vi "LSMcontroller_v57.vi"() -> ()   [LabVIEW 2015] (continued)
                n2498 = property on="Sampling rate" class="DigNum (strict)"("Visible"=FALSE, "DisabledEnum"=T8."Disabled" ("Disabled")) -> ()  [unwired: 2 in, 2 out]
                n2499 = property on="Pel" class="DigNum (strict)"("Visible"=w5442, "DisabledEnum"=w5443) -> ()  [unwired: 2 in, 2 out]
                n2500 = property on="bin" class="DigNum (strict)"("Visible"=w5442, "DisabledEnum"=w5443) -> ()  [unwired: 2 in, 2 out]
                n2501 = call "2pparameters.vi"("Params in"=w5453, "command"="set") -> ()  [unwired: 1 out]
              }
              frame "Lifetime (point)" {
                w5476 = T8."Enabled" ("Disabled")
                w5475 = TRUE ("Visible")
                n2502 = property on="Pel" class="DigNum (strict)"("Visible"=w5475, "DisabledEnum"=w5476) -> ()  [unwired: 2 in, 2 out]
                n2503 = property on="bin" class="DigNum (strict)"("Visible"=w5475, "DisabledEnum"=w5476) -> ()  [unwired: 2 in, 2 out]
                n2504 = property on="ttt" class="Enum (strict)"("Visible"=FALSE) -> ()  [unwired: 2 in, 2 out]
                n2505 = local write "Zscantab"(enum32{"withzscan", "withoutzscan", "lifetime"}."lifetime" ("Zscantab")) -> ()
                n2506 = local write "graphtab"(T6."Lifetime" ("graphtab")) -> ()
                n2507 = local write "Meastab"(enum32{"X-Y Image", "Linescan", "Timetrace"}."Timetrace" ("Meastab")) -> ()
                n2508 = call "lifetimeparameters.vi"("command"="get") -> ("Params out"=w5483:T21)  [unwired: 1 in]
                n2509 = Unbundle By Name(w5483) -> ("initialized"=w5484:bool)
                n2510 = property on="srateAODOtt" class="DigNum (strict)"("Visible"=TRUE, "DisabledEnum"=T8."Enabled" ("Disabled")) -> ()  [unwired: 2 in, 2 out]
                n2511 = case shown="False" w5484 {
                  frame False {
                    n2512 = property on="Init" class="Bool (strict)"("Visible"=TRUE, "DisabledEnum"=T8."Enabled" ("Disabled")) -> ()  [unwired: 2 in, 2 out]
                    n2513 = property on="Start" class="Bool (strict)"("Visible"=FALSE, "DisabledEnum"=T8."Disabled and Grayed Out" ("Disabled")) -> ()  [unwired: 2 in, 2 out]
                  }
                  frame True {
                  }
                }
                n2514 = property on="Sampling rate" class="DigNum (strict)"("Visible"=FALSE, "DisabledEnum"=T8."Disabled" ("Disabled")) -> ()  [unwired: 2 in, 2 out]
              }
              frame "Lifetime (scan)" {
                w5493 = T8."Disabled" ("Disabled")
                w5492 = FALSE ("Visible")
                n2515 = call "lifetimeparameters.vi"("command"="get") -> ("Params out"=w5505:T21)  [unwired: 1 in]
                n2516 = local write "graphtab"(T6."image" ("graphtab")) -> ()
                n2517 = local write "Save tab"(enum32{"withsave", "withoutsave"}."withsave" ("Save tab")) -> ()
                n2518 = local write "Meastab"(enum32{"X-Y Image", "Linescan", "Timetrace"}."X-Y Image" ("Meastab")) -> ()
                n2519 = local write "Zscantab"(enum32{"withzscan", "withoutzscan", "lifetime"}."lifetime" ("Zscantab")) -> ()
                n2520 = Unbundle By Name(w5505) -> ("initialized"=w5504:bool)
                n2521 = property on="ttt" class="Enum (strict)"("Visible"=FALSE) -> ()  [unwired: 2 in, 2 out]
                n2522 = property on="refreshtime" class="DigNum (strict)"("Visible"=FALSE, "DisabledEnum"=T8."Disabled and Grayed Out" ("Disabled")) -> ()  [unwired: 2 in, 2 out]
                n2523 = property on="Pel" class="DigNum (strict)"("Visible"=w5492, "DisabledEnum"=w5493) -> ()  [unwired: 2 in, 2 out]
                n2524 = property on="bin" class="DigNum (strict)"("Visible"=w5492, "DisabledEnum"=w5493) -> ()  [unwired: 2 in, 2 out]
                n2525 = property on="save data" class="Bool (strict)"("Visible"=TRUE, "DisabledEnum"=T8."Enabled" ("Disabled"), "Value"=TRUE ("Visible")) -> ()  [unwired: 2 in, 2 out]
                n2526 = case shown="False" w5504 {
                  frame False {
                    n2527 = property on="Init" class="Bool (strict)"("Visible"=TRUE, "DisabledEnum"=T8."Enabled" ("Disabled")) -> ()  [unwired: 2 in, 2 out]
                    n2528 = property on="Start" class="Bool (strict)"("Visible"=FALSE, "DisabledEnum"=T8."Disabled and Grayed Out" ("Disabled")) -> ()  [unwired: 2 in, 2 out]
                  }
                  frame True {
                  }
                }
                n2529 = call "2pparameters.vi"("command"="get") -> ("params out"=w5510:T12)  [unwired: 1 in]
                n2530 = property on="continuous" class="Bool (strict)"("Visible"=TRUE, "DisabledEnum"=T8."Disabled and Grayed Out" ("Disabled")) -> ()  [unwired: 2 in, 2 out]
                n2531 = property on="finite samples" class="Bool (strict)"("Visible"=TRUE, "DisabledEnum"=T8."Enabled" ("Disabled")) -> ()  [unwired: 2 in, 2 out]
                n2532 = Bundle By Name(cluster=w5510, "type"="Lifetime (scan)") -> (w5508:T12)
                n2533 = call "2pparameters.vi"("Params in"=w5508, "command"="set") -> ()  [unwired: 1 out]
                n2534 = property on="finite samples" class="Bool (strict)"("Val(Sgnl)"=TRUE ("continuous for display")) -> ()  [unwired: 2 in, 2 out]
                n2535 = property on="continuous" class="Bool (strict)"("Value"=FALSE ("continuous for display")) -> ()  [unwired: 2 in, 2 out]
                n2536 = property on="srateAODOtt" class="DigNum (strict)"("Visible"=FALSE, "DisabledEnum"=T8."Disabled" ("Disabled")) -> ()  [unwired: 2 in, 2 out]
                n2537 = property on="# of frames" class="DigNum (strict)"("DisabledEnum"=T8."Enabled" ("Disabled"), "Caption.Text"="# of frames") -> ()  [unwired: 2 in, 2 out]
                n2538 = property on="img_CH1" class="IntGraph (strict)"("ZScale.Maximum"=12.5 ("Z Scale.Range:Maximum")) -> ()  [unwired: 2 in, 2 out]
                n2539 = property on="Current Average" class="DigNum (strict)"("Visible"=TRUE, "DisabledEnum"=T8."Enabled" ("Disabled")) -> ()  [unwired: 2 in, 2 out]
                n2540 = property on="Sampling rate" class="DigNum (strict)"("Visible"=TRUE, "DisabledEnum"=T8."Enabled" ("Disabled")) -> ()  [unwired: 2 in, 2 out]
                n2541 = property on="avpp" class="DigNum (strict)"("Visible"=TRUE, "DisabledEnum"=T8."Enabled" ("Disabled")) -> ()  [unwired: 2 in, 2 out]
              }
              frame "Lifetime (contour)" {
                w5534 = T8."Enabled" ("Disabled")
                w5533 = TRUE ("Visible")
                n2542 = call "2pparameters.vi"("command"="get") -> ("params out"=w5541:T12)  [unwired: 1 in]
                n2543 = property on="# of frames" class="DigNum (strict)"("DisabledEnum"=T8."Enabled" ("Disabled"), "Caption.Text"="# of samples") -> ()  [unwired: 2 in, 2 out]
                n2544 = property on="refreshtime" class="DigNum (strict)"("Visible"=TRUE, "DisabledEnum"=T8."Enabled" ("Disabled")) -> ()  [unwired: 2 in, 2 out]
                n2545 = Unbundle By Name(w5541) -> ("Angle draw"=w5543:dbl)
                n2546 = property on="avpp" class="DigNum (strict)"("Visible"=FALSE, "DisabledEnum"=T8."Disabled and Grayed Out" ("Disabled")) -> ()  [unwired: 2 in, 2 out]
                n2547 = property on="Current Average" class="DigNum (strict)"("Visible"=FALSE, "DisabledEnum"=T8."Disabled and Grayed Out" ("Disabled")) -> ()  [unwired: 2 in, 2 out]
                n2548 = local write "Angle drawing"(w5543) -> ()
                n2549 = local write "Save tab"(enum32{"withsave", "withoutsave"}."withsave" ("Save tab")) -> ()
                n2550 = local write "Zscantab"(enum32{"withzscan", "withoutzscan", "lifetime"}."lifetime" ("Zscantab")) -> ()
                n2551 = local write "graphtab"(T6."Lifetime" ("graphtab")) -> ()
                n2552 = local write "Meastab"(enum32{"X-Y Image", "Linescan", "Timetrace"}."Timetrace" ("Meastab")) -> ()
                n2553 = property on="ttt" class="Enum (strict)"("Visible"=TRUE) -> ()  [unwired: 2 in, 2 out]
                n2554 = call "lifetimeparameters.vi"("command"="get") -> ("Params out"=w5565:T21)  [unwired: 1 in]
                n2555 = property on="finite samples" class="Bool (strict)"("Val(Sgnl)"=TRUE ("continuous for display")) -> ()  [unwired: 2 in, 2 out]
                n2556 = local write "save\ndata"(TRUE ("save\ndata")) -> ()
                n2557 = Unbundle By Name(w5565) -> ("initialized"=w5566:bool)
                n2558 = property on="continuous" class="Bool (strict)"("Visible"=TRUE, "DisabledEnum"=T8."Enabled" ("Disabled")) -> ()  [unwired: 2 in, 2 out]
                n2559 = property on="finite samples" class="Bool (strict)"("Visible"=TRUE, "DisabledEnum"=T8."Enabled" ("Disabled")) -> ()  [unwired: 2 in, 2 out]
                n2560 = property on="Pel" class="DigNum (strict)"("Visible"=w5533, "DisabledEnum"=w5534) -> ()  [unwired: 2 in, 2 out]
                n2561 = property on="bin" class="DigNum (strict)"("Visible"=w5533, "DisabledEnum"=w5534) -> ()  [unwired: 2 in, 2 out]
                n2562 = property on="continuous" class="Bool (strict)"("Value"=FALSE ("continuous for display")) -> ()  [unwired: 2 in, 2 out]
                n2563 = case shown="False" w5566 {
                  frame False {
                    n2564 = property on="Init" class="Bool (strict)"("Visible"=TRUE, "DisabledEnum"=T8."Enabled" ("Disabled")) -> ()  [unwired: 2 in, 2 out]
                    n2565 = property on="Start" class="Bool (strict)"("Visible"=FALSE, "DisabledEnum"=T8."Disabled and Grayed Out" ("Disabled")) -> ()  [unwired: 2 in, 2 out]
                  }
                  frame True {
                  }
                }
                n2566 = property on="srateAODOtt" class="DigNum (strict)"("Visible"=TRUE, "DisabledEnum"=T8."Enabled" ("Disabled")) -> ()  [unwired: 2 in, 2 out]
                n2567 = call "2pparameters.vi"("command"="get") -> ("params out"=w5545:T12)  [unwired: 1 in]
                n2568 = Bundle By Name(cluster=w5545, "type"="Timetrace") -> (w5539:T12)
                n2569 = call "2pparameters.vi"("Params in"=w5539, "command"="set") -> ()  [unwired: 1 out]
                n2570 = property on="Sampling rate" class="DigNum (strict)"("Visible"=FALSE, "DisabledEnum"=T8."Disabled" ("Disabled")) -> ()  [unwired: 2 in, 2 out]
              }
            }
          }
          event "Laserpower \n(%)": Value Change {
            n2571 = event-data() -> ("OldVal"=w5574:dbl, "NewVal"=w5575:dbl)  [unwired: 1 in, 4 out]
            n2572 = Not Equal?(x=w5574, y=w5575) -> (x != y?=w5576:bool)
            n2573 = case shown="True" w5576 {
              tunnel: w5575 -> [_ w5577]
              frame False {
              }
              frame True {
                n2574 = local read "wavelength(nm)"() -> (w5579:dbl)
                n2575 = call "configuration.vi"("command"="get") -> ("config out"=w5583:T13)  [unwired: 2 in, 1 out]
                n2576 = call "pockelscellcalibration.vi"("l"=w5579, "T"=w5577) -> ("Vout"=w5578:dbl)
                n2577 = Unbundle By Name(w5583) -> ("Vto2P"=w5582:i32, "AOlines"=w5581:tag[])
                n2578 = property on="lpow" class="DigNum (strict)"("Value"=w5577) -> ()  [unwired: 2 in, 2 out]
                n2579 = Index Array(array=w5581, index=w5582) -> (element=w5580:tag)
                n2580 = call-poly <vilib>:"DAQmx Create Virtual Channel.vi"("physical channels"=w5580) -> ("task out"=w5586:refnum<k21>, "error out"=w5585:errorcluster)  [unwired: 13 in]
                n2581 = call-poly <vilib>:"DAQmx Write.vi"("task/channels in"=w5586, "data"=w5578, "error in"=w5585) -> ("task out"=w5587:refnum<k21>, "error out"=w5588:errorcluster)  [unwired: 10 in, 1 out]
                n2582 = call <vilib>:"DAQmx Start Task.vi"("task/channels in"=w5587, "error in"=w5588) -> ("task out"=w5589:refnum<k21>, "error out"=w5590:errorcluster)  [unwired: 12 in]
                n2583 = call <vilib>:"DAQmx Stop Task.vi"("task/channels in"=w5589, "error in"=w5590) -> ("task out"=w5591:refnum<k21>, "error out"=w5592:errorcluster)  [unwired: 12 in]
                n2584 = call <vilib>:"DAQmx Clear Task.vi"("task in"=w5591, "error in"=w5592) -> ()  [unwired: 13 in, 1 out]
              }
            }
          }
          event "lpow": Value Change {
            n2585 = event-data() -> ("OldVal"=w5593:dbl, "NewVal"=w5594:dbl)  [unwired: 1 in, 4 out]
            n2586 = Not Equal?(x=w5593, y=w5594) -> (x != y?=w5595:bool)
            n2587 = case shown="True" w5595 {
              tunnel: w5594 -> [_ w5598]
              frame False {
              }
              frame True {
                n2588 = local read "wavelength(nm)"() -> (w5597:dbl)
                n2589 = call "pockelscellcalibration.vi"("l"=w5597, "T"=w5598) -> ("Vout"=w5596:dbl)
                n2590 = call "configuration.vi"("command"="get") -> ("config out"=w5602:T13)  [unwired: 2 in, 1 out]
                n2591 = Unbundle By Name(w5602) -> ("Vto2P"=w5601:i32, "AOlines"=w5600:tag[])
                n2592 = property on="Laserpower \n(%)" class="Slide (strict)"("Value"=w5598) -> ()  [unwired: 2 in, 2 out]
                n2593 = Index Array(array=w5600, index=w5601) -> (element=w5599:tag)
                n2594 = call-poly <vilib>:"DAQmx Create Virtual Channel.vi"("physical channels"=w5599) -> ("task out"=w5605:refnum<k21>, "error out"=w5604:errorcluster)  [unwired: 13 in]
                n2595 = call-poly <vilib>:"DAQmx Write.vi"("task/channels in"=w5605, "data"=w5596, "error in"=w5604) -> ("task out"=w5606:refnum<k21>, "error out"=w5607:errorcluster)  [unwired: 10 in, 1 out]
                n2596 = call <vilib>:"DAQmx Start Task.vi"("task/channels in"=w5606, "error in"=w5607) -> ("task out"=w5608:refnum<k21>, "error out"=w5609:errorcluster)  [unwired: 12 in]
                n2597 = call <vilib>:"DAQmx Stop Task.vi"("task/channels in"=w5608, "error in"=w5609) -> ("task out"=w5610:refnum<k21>, "error out"=w5611:errorcluster)  [unwired: 12 in]
                n2598 = call <vilib>:"DAQmx Clear Task.vi"("task in"=w5610, "error in"=w5611) -> ()  [unwired: 13 in, 1 out]
              }
            }
          }
          event "sealtest": Value Change {
            n2599 = event-data() -> ()  [unwired: 1 in, 6 out]
            n2600 = case shown="True" "sealtest" {
              frame False {
              }
              frame True {
                n2601 = stacked-sequence {
                  seq-local: [w5613 _ _ _ _ _] -> [_ w5646 _ w5698 _ _]
                  frame #0 {
                    n2602 = stacked-sequence {
                      tunnel: [_ w5625 _] -> w5613
                      frame #0 {
                        n2603 = call "2pparameters.vi"("command"="get") -> ("params out"=w5618:T12)  [unwired: 1 in]
                        n2604 = Unbundle By Name(w5618) -> ("autoshutter"=w5619:bool)
                        n2605 = local read "OCchecked?"() -> (w5616:bool)
                        n2606 = call "sealtestwfparams.vi"("command"="set") -> ()  [unwired: 6 in, 1 out]
                        n2607 = case shown="False" w5616 {
                          frame False {
                            n2608 = One Button Dialog(message="Is the OC gain correct?", button name ("OK")="ok") -> (true=w5620:bool)
                            n2609 = local write "OCchecked?"(w5620) -> ()
                          }
                          frame True {
                          }
                        }
                        n2610 = case shown="True" w5619 {
                          frame False {
                          }
                          frame True {
                            n2611 = call "shuttercontrol.vi"("command"="close") -> ()  [unwired: 1 in, 1 out]
                          }
                        }
                        n2612 = call "allAI-temp.vi"("command"=enum16{"get", "set", "clear", "append"}."clear") -> ()  [unwired: 3 in, 2 out]
                      }
                      frame #1 {
                        n2613 = call "sealtestwfparams.vi"("command"="get") -> ("Params out"=w5631:T25)  [unwired: 6 in]
                        n2614 = Unbundle By Name(w5631) -> ("AO parameters"=w5629:T1)
                        "AO parameters 2" <- w5629
                        n2615 = Index Array(array=w5629, index=0) -> (element=w5628:T26)
                        n2616 = call "generateRampedSquareWave_fromAOparameters.vi"("AO params"=w5628) -> ("Waveform"=w5624:waveform(dbl), "wflength"=w5625:i32)
                        "Waveform Graph" <- w5624
                        "wflength" <- w5625
                        n2617 = Build Array(w5624) -> (w5627:waveform(dbl)[])
                        n2618 = call "waveformssealtestbuffer.vi"("AO wf in"=w5627, "command"="set") -> ()  [unwired: 1 out]
                      }
                      frame #2 {
                        n2619 = local read "Vholding (mV)"() -> (w5634:sgl)
                        n2620 = local read "Current Clamp"() -> (w5640:bool)
                        n2621 = local read "Voltage Clamp"() -> (w5639:bool)
                        n2622 = local read "OCgain"() -> (w5635:sgl)
                        n2623 = local read "CC_ICgain"() -> (w5638:dbl)
                        n2624 = local read "holdon"() -> (w5633:bool)
                        n2625 = call "patchparameters.vi"("command"="get") -> ("Params out"=w5642:T15)  [unwired: 1 in]
                        n2626 = Bundle By Name(cluster=w5642, "VC"=w5639, "CC"=w5640, "CC_icg (pA/mv)"=w5638, "VC_icg (mV/mV)"=10.0, "OCG (mV/pA)"=w5635, "OVG (mV/mV)"=0.1, "Vhold (mV)"=w5634, "holdon"=w5633) -> (w5641:T15)
                        n2627 = call "patchparameters.vi"("Params in"=w5641, "command"="set") -> ()  [unwired: 1 out]
                      }
                    }
                  }
                  frame #1 {
                    w5645 = 2
                    n2628 = call "patchparameters.vi"("command"="get") -> ("Params out"=w5653:T15)  [unwired: 1 in]
                    n2629 = Unbundle By Name(w5653) -> ("holdon"=w5652:bool, "Vhold (mV)"=w5651:sgl, "CC_icg (pA/mv)"=w5659:sgl, "CC"=w5657:bool, "VC_icg (mV/mV)"=w5658:sgl)
                    n2630 = Select(t=w5659, s=w5657, f=w5658) -> (s? t:f=w5660:sgl)
                    n2631 = To Single Precision Float(number=0.001 ("y")) -> (single precision float=w5661:sgl)
                    n2632 = Compound Arithmetic op=MULTIPLY(w5651, w5660, w5661) -> (w5655:sgl)
                    n2633 = case shown="False" w5652 {
                      tunnel: w5655 -> [_ w5673]
                      tunnel: [0.0 w5673] -> w5648
                      frame False {
                      }
                      frame True {
                      }
                    }
                    n2634 = Greater Than 0?(x=w5645) -> (x > 0?=w5647:bool)
                    n2635 = case shown="True" w5647 {
                      tunnel: w5646 -> [_ w5662]
                      tunnel: w5645 -> [_ w5665]
                      frame False {
                      }
                      frame True {
                        n2636 = Initialize Array(sgl 0.0 ("element"), w5665, w5662) -> (w5663:sgl[][])
                        n2637 = call "allAI-temp.vi"("array in"=w5663, "command"=enum16{"get", "set", "clear", "append"}."set") -> ()  [unwired: 2 in, 2 out]
                      }
                    }
                    n2638 = flat-sequence {
                      tunnel: w5646 -> [w5669]
                      tunnel: w5646 -> [w5668]
                      tunnel: [w5668] -> w5650
                      tunnel: [w5667] -> w5649
                      tunnel: w5648 -> [w5667]
                      tunnel: w5650 -> [w5671]
                      tunnel: w5649 -> [w5670]
                      frame #0 {
                        n2639 = call "prepAI_sealtest.vi"("samples per channel"=w5669) -> ()  [unwired: 2 in]
                      }
                      frame #1 {
                        n2640 = call "prepAO_sealtest.vi"("Vhold"=w5670, "samples per channel"=w5671) -> ()  [unwired: 1 in]
                      }
                    }
                  }
                  frame #2 {
                    n2641 = stacked-sequence {
                      frame #0 {
                        n2642 = call "tempconfigAO.vi"("command"="get") -> ("Temp Config out"=w5677:T27)  [unwired: 1 in]
                        n2643 = Unbundle By Name(w5677) -> ("AO"=w5678:refnum<k21>[], "E_AO"=w5679:errorcluster[])
                        n2644 = for {
                          tunnel: w5678 -> [w5687] mode=indexing
                          tunnel: w5679 -> [w5686] mode=indexing
                          tunnel: [w5685] -> w5681 mode=indexing
                          tunnel: [w5684] -> w5682 mode=indexing
                          n2645 = call <vilib>:"DAQmx Start Task.vi"("task/channels in"=w5687, "error in"=w5686) -> ("task out"=w5685:refnum<k21>, "error out"=w5684:errorcluster)  [unwired: 12 in]
                        }
                        n2646 = call "tempconfigAO.vi"("command"="get") -> ("Temp Config out"=w5680:T27)  [unwired: 1 in]
                        n2647 = Bundle By Name(cluster=w5680, "AO"=w5681, "E_AO"=w5682) -> (w5683:T27)
                        n2648 = call "tempconfigAO.vi"("Temp Config in"=w5683, "command"="set") -> ()  [unwired: 1 out]
                      }
                      frame #1 {
                        n2649 = call "tempconfigAI.vi"("command"="get") -> ("Temp Config out"=w5689:T28)  [unwired: 1 in]
                        n2650 = Unbundle By Name(w5689) -> ("AI"=w5694:refnum<k21>, "E_AI"=w5695:errorcluster)
                        n2651 = call <vilib>:"DAQmx Start Task.vi"("task/channels in"=w5694, "error in"=w5695) -> ("task out"=w5696:refnum<k21>, "error out"=w5697:errorcluster)  [unwired: 12 in]
                        n2652 = call "tempconfigAI.vi"("command"="get") -> ("Temp Config out"=w5691:T28)  [unwired: 1 in]
                        n2653 = Bundle By Name(cluster=w5691, "AI"=w5696, "E_AI"=w5697) -> (w5693:T28)
                        n2654 = call "tempconfigAI.vi"("Temp Config in"=w5693, "command"="set") -> ()  [unwired: 1 out]
                      }
                    }
                  }
                  frame #3 {
                    n2655 = while {
                      tunnel: w5698 -> [w5699]
                      stop <- w5700 stop-if-true
                      n2656 = local read "sealtest"() -> (w5703:bool)
                      n2657 = Not(x=w5703) -> (.not. x?=w5702:bool)
                      n2658 = case shown="False" w5702 {
                        tunnel: w5699 -> [w5704 _]
                        frame False {
                          n2659 = stacked-sequence {
                            seq-local: [_ _ _ w5743 _ _] -> [_ _ _ _ w5799 _]
                            seq-local: [w5705 _ _ _ _ _] -> [_ w5714 _ w5736 w5788 w5819]
                            tunnel: w5704 -> [_ _ w5722 _ w5787 _]
                            frame #0 {
                              n2660 = call "patchparameters.vi"("command"="get") -> ("Params out"=w5712:T15)  [unwired: 1 in]
                              n2661 = local read "Vholding (mV)"() -> (w5709:sgl)
                              n2662 = Unbundle By Name(w5712) -> ("Vhold (mV)"=w5708:sgl, "holdon"=w5711:bool)
                              n2663 = local read "holdon"() -> (w5710:bool)
                              n2664 = Not Equal?(x=w5709, y=w5708) -> (x != y?=w5707:bool)
                              n2665 = Not Equal?(x=w5711, y=w5710) -> (x != y?=w5706:bool)
                              n2666 = Or(x=w5707, y=w5706) -> (x .or. y?=w5705:bool)
                            }
                            frame #1 {
                              n2667 = case shown="True" w5714 {
                                frame False {
                                }
                                frame True {
                                n2668 = local read "Vholding (mV)"() -> (w5717:sgl)
                                n2669 = local read "holdon"() -> (w5715:bool)
                                n2670 = call "patchparameters.vi"("command"="get") -> ("Params out"=w5718:T15)  [unwired: 1 in]
                                n2671 = Bundle By Name(cluster=w5718, "Vhold (mV)"=w5717, "holdon"=w5715) -> (w5716:T15)
                                n2672 = call "patchparameters.vi"("Params in"=w5716, "command"="set") -> ()  [unwired: 1 out]
                                }
                              }
                            }
                            frame #2 {
                              n2673 = call "tempconfigAI.vi"("command"="get") -> ("Temp Config out"=w5732:T28)  [unwired: 1 in]
                              n2674 = Unbundle By Name(w5732) -> ("AI"=w5731:refnum<k21>, "E_AI"=w5730:errorcluster)
                              n2675 = call-poly <vilib>:"DAQmx Read.vi"("task/channels in"=w5731, "number of samples per channel"=w5722, "timeout"=10.0, "error in"=w5730) -> ("task out"=w5726:refnum<k21>, "data"=w5723:i16[][], "error out"=w5735:errorcluster)  [unwired: 9 in]
                              n2676 = call "tempconfigAI.vi"("command"="get") -> ("Temp Config out"=w5727:T28)  [unwired: 1 in]
                              n2677 = Bundle By Name(cluster=w5727, "AI"=w5726, "E_AI"=w5735) -> (w5734:T28)
                              n2678 = To Single Precision Float(number=w5723) -> (single precision float=w5725:sgl[][])
                              n2679 = call "tempconfigAI.vi"("Temp Config in"=w5734, "command"="set") -> ()  [unwired: 1 out]
                              n2680 = call "allAI-temp.vi"("array in"=w5725, "command"=enum16{"get", "set", "clear", "append"}."set") -> ()  [unwired: 2 in, 2 out]
                            }
                            frame #3 {
                              n2681 = case shown="True" w5736 {
                                frame False {
                                }
                                frame True {
                                n2682 = call "tempconfigAO.vi"("command"="get") -> ("Temp Config out"=w5776:T27)  [unwired: 1 in]
                                n2683 = Unbundle By Name(w5776) -> ("AO"=w5775:refnum<k21>[], "E_AO"=w5774:errorcluster[])
                                n2684 = call "tempconfigAI.vi"("command"="get") -> ("Temp Config out"=w5763:T28)  [unwired: 1 in]
                                n2685 = Unbundle By Name(w5763) -> ("AI"=w5764:refnum<k21>, "E_AI"=w5765:errorcluster)
                                n2686 = for {
                                tunnel: w5775 -> [w5780] mode=indexing
                                tunnel: w5774 -> [w5779] mode=indexing
                                tunnel: [w5778] -> w5770 mode=indexing
                                n2687 = call <vilib>:"DAQmx Stop Task.vi"("task/channels in"=w5780, "error in"=w5779) -> ("task out"=w5781:refnum<k21>, "error out"=w5782:errorcluster)  [unwired: 12 in]
                                n2688 = call <vilib>:"DAQmx Clear Task.vi"("task in"=w5781, "error in"=w5782) -> ("error out"=w5778:errorcluster)  [unwired: 13 in]
                                }
                                n2689 = call <vilib>:"DAQmx Stop Task.vi"("task/channels in"=w5764, "error in"=w5765) -> ("task out"=w5761:refnum<k21>, "error out"=w5760:errorcluster)  [unwired: 12 in]
                                n2690 = call <vilib>:"DAQmx Clear Task.vi"("task in"=w5761, "error in"=w5760) -> ("error out"=w5759:errorcluster)  [unwired: 13 in]
                                n2691 = call "tempconfigAO.vi"("command"="get") -> ("Temp Config out"=w5771:T27)  [unwired: 1 in]
                                n2692 = Bundle By Name(cluster=w5771, "E_AO"=w5770) -> (w5769:T27)
                                n2693 = call "tempconfigAI.vi"("command"="get") -> ("Temp Config out"=w5767:T28)  [unwired: 1 in]
                                n2694 = Bundle By Name(cluster=w5767, "E_AI"=w5759) -> (w5758:T28)
                                n2695 = call "tempconfigAO.vi"("Temp Config in"=w5769, "command"="set") -> ()  [unwired: 1 out]
                                n2696 = call "tempconfigAI.vi"("Temp Config in"=w5758, "command"="set") -> ()  [unwired: 1 out]
                                }
                              }
                              n2697 = call "allAI-temp.vi"("command"=enum16{"get", "set", "clear", "append"}."get") -> ("array out"=w5740:sgl[][])  [unwired: 3 in, 1 out]
                              n2698 = call "tempconfigAI.vi"("command"="get") -> ("Temp Config out"=w5753:T28)  [unwired: 1 in]
                              n2699 = call "tempconfigAI.vi"("command"="get") -> ("Temp Config out"=w5755:T28)  [unwired: 1 in]
                              n2700 = Unbundle By Name(w5753) -> ("header"=w5751:dbl[])
                              n2701 = Unbundle By Name(w5755) -> ("header"=w5757:dbl[])
                              n2702 = Index Array(array=w5740, index (row) #1=1 ("index (row)"), index (row) #2=0 ("index (row)")) -> (element #1=w5738:sgl[], element #2=w5737:sgl[])  [unwired: 2 in]
                              n2703 = local read "OCgain"() -> (w5745:sgl)
                              n2704 = call "Unscaledtoscaled.vi"("Unscaled Data"=w5738, "Header Information"=w5751) -> ("Array"=w5750:sgl[])  [unwired: 1 in]
                              n2705 = call "Unscaledtoscaled.vi"("Unscaled Data"=w5737, "Header Information"=w5757) -> ("Array"=w5754:sgl[])  [unwired: 1 in]
                              n2706 = Multiply(x=w5750, y=0.1) -> (x*y=w5747:dbl[])
                              n2707 = Divide(x=w5754, y=w5745) -> (x/y=w5746:sgl[])
                              n2708 = Build Array(w5747, w5746) -> (w5749:dbl[][])
                              n2709 = Multiply(x=w5749, y=1000.0) -> (x*y=w5743:dbl[][])
                              "Patch readout" <- w5743
                            }
                            frame #4 {
                              n2710 = case shown="True" w5788 {
                                tunnel: w5787 -> [_ w5800]
                                frame False {
                                }
                                frame True {
                                n2711 = call "patchparameters.vi"("command"="get") -> ("Params out"=w5804:T15)  [unwired: 1 in]
                                n2712 = Unbundle By Name(w5804) -> ("holdon"=w5803:bool, "Vhold (mV)"=w5802:sgl, "CC_icg (pA/mv)"=w5810:sgl, "CC"=w5808:bool, "VC_icg (mV/mV)"=w5809:sgl)
                                n2713 = Select(t=w5810, s=w5808, f=w5809) -> (s? t:f=w5811:sgl)
                                n2714 = To Single Precision Float(number=0.001 ("y")) -> (single precision float=w5812:sgl)
                                n2715 = Compound Arithmetic op=MULTIPLY(w5802, w5811, w5812) -> (w5806:sgl)
                                n2716 = case shown="True" w5803 {
                                tunnel: w5806 -> [_ w5817]
                                tunnel: [0.0 w5817] -> w5801
                                frame False {
                                }
                                frame True {
                                }
                                }
                                n2717 = flat-sequence {
                                tunnel: w5800 -> [w5813]
                                tunnel: w5801 -> [w5815]
                                tunnel: w5800 -> [w5814]
                                frame #0 {
                                n2718 = call "prepAI_sealtest.vi"("samples per channel"=w5813) -> ()  [unwired: 2 in]
                                }
                                frame #1 {
                                n2719 = call "prepAO_sealtest.vi"("Vhold"=w5815, "samples per channel"=w5814) -> ()  [unwired: 1 in]
                                }
                                }
                                }
                              }
                              n2720 = call "sealtestwfparams.vi"("command"="get") -> ("Params out"=w5793:T25)  [unwired: 6 in]
                              n2721 = Unbundle By Name(w5793) -> ("AO parameters"=w5794:T1)
                              n2722 = Index Array(array=w5794, index=0) -> (element=w5796:T26)
                              n2723 = Unbundle By Name(w5796) -> ("Cycles"=w5791:dbl, "Start amplitude (V)"=w5790:dbl, "Sampling frequency (Hz)"=w5789:dbl)
                              n2724 = local read "fitpoints"() -> (w5797:dbl)
                              n2725 = script code="V=data(1,:);\nI=data(2,:);\ntres=mean(V);\nspc=(nsamp./ncyc);\nV=V(spc+1:end-spc);\nI=I(spc+1:end-spc);\ndV=mean(V(V>tres))-mean(V(V<tres))\nIcyc=reshape(I,[spc ncyc-2]);\nIcyc=Icyc';\nIcyc=mean(Icyc,1);\ndIss=mean(Icyc(floor(spc*0.15):floor(spc/2)-2))-mean(Icyc(spc*0.65:spc-2))\nRm=dV*1e3/dIss;\n[maxi,ind]=max(Icyc);\nIfit=Icyc(ind+1:ind+1+points-1)-0.5*(mean(Icyc(floor(spc*0.15):floor(spc/2)-2))+mean(Icyc(spc*0.65:spc-2)))\nt=(3:points-1+3)./srate*1000;\nt=t';\nIfit=Ifit';\nc=fit(t,Ifit, 'exp1');\ncoeffs=coeffvalues(c);\nIa=coeffs(1);\nRa=dV*1e3./Ia/2;\ntau=-1./coeffs(2);\ncap=tau/Ra*1000;"("data"=w5799, "nsamp"=w5787, "ncyc"=w5791, "maxV"=w5790, "points"=w5797, "srate"=w5789) -> ("cap"=w5786:dbl, "Ra"=w5785:dbl, "Icyc"=w5784:dbl[], "Rm"=w5783:dbl)  [unwired: 1 in, 1 out]
                              n2726 = local read "set as Rp?"() -> (w5798:bool)
                              n2727 = local write "Cmembrane"(w5786) -> ()
                              n2728 = local write "Rmembrane (MOhm)"(w5783) -> ()
                              n2729 = local write "Racces (MOhm)"(w5785) -> ()
                              n2730 = case shown="True" w5798 {
                                tunnel: w5783 -> [_ w5818]
                                frame False {
                                }
                                frame True {
                                n2731 = local write "Rpipette (MOhm)"(w5818) -> ()
                                }
                              }
                              n2732 = local write "Ifit"(w5784) -> ()
                            }
                            frame #5 {
                              n2733 = local read "set as Rp?"() -> (w5820:bool)
                              n2734 = case shown="True" w5819 {
                                frame False {
                                }
                                frame True {
                                n2735 = stacked-sequence {
                                frame #0 {
                                n2736 = call "tempconfigAO.vi"("command"="get") -> ("Temp Config out"=w5827:T27)  [unwired: 1 in]
                                n2737 = Unbundle By Name(w5827) -> ("AO"=w5826:refnum<k21>[], "E_AO"=w5825:errorcluster[])
                                n2738 = for {
                                tunnel: w5826 -> [w5834] mode=indexing
                                tunnel: w5825 -> [w5833] mode=indexing
                                tunnel: [w5832] -> w5823 mode=indexing
                                tunnel: [w5831] -> w5822 mode=indexing
                                n2739 = call <vilib>:"DAQmx Start Task.vi"("task/channels in"=w5834, "error in"=w5833) -> ("task out"=w5832:refnum<k21>, "error out"=w5831:errorcluster)  [unwired: 12 in]
                                }
                                n2740 = call "tempconfigAO.vi"("command"="get") -> ("Temp Config out"=w5824:T27)  [unwired: 1 in]
                                n2741 = Bundle By Name(cluster=w5824, "AO"=w5823, "E_AO"=w5822) -> (w5821:T27)
                                n2742 = call "tempconfigAO.vi"("Temp Config in"=w5821, "command"="set") -> ()  [unwired: 1 out]
                                }
                                frame #1 {
                                n2743 = call "tempconfigAI.vi"("command"="get") -> ("Temp Config out"=w5836:T28)  [unwired: 1 in]
                                n2744 = Unbundle By Name(w5836) -> ("AI"=w5841:refnum<k21>, "E_AI"=w5842:errorcluster)
                                n2745 = call <vilib>:"DAQmx Start Task.vi"("task/channels in"=w5841, "error in"=w5842) -> ("task out"=w5843:refnum<k21>, "error out"=w5844:errorcluster)  [unwired: 12 in]
                                n2746 = call "tempconfigAI.vi"("command"="get") -> ("Temp Config out"=w5838:T28)  [unwired: 1 in]
                                n2747 = Bundle By Name(cluster=w5838, "AI"=w5843, "E_AI"=w5844) -> (w5840:T28)
                                n2748 = call "tempconfigAI.vi"("Temp Config in"=w5840, "command"="set") -> ()  [unwired: 1 out]
                                }
                                }
                                }
                              }
                              n2749 = case shown="True" w5820 {
                                frame False {
                                }
                                frame True {
                                n2750 = local write "set as Rp?"(FALSE ("set as Rp?")) -> ()
                                }
                              }
                            }
                          }
                        }
                        frame True {
                        }
                      }
                      n2751 = local read "sealtest"() -> (w5701:bool)
                      n2752 = Not(x=w5701) -> (.not. x?=w5700:bool)
                    }
                  }
                  frame #4 {
                    n2753 = call "tempconfigAO.vi"("command"="get") -> ("Temp Config out"=w5871:T27)  [unwired: 1 in]
                    n2754 = Unbundle By Name(w5871) -> ("AO"=w5870:refnum<k21>[], "E_AO"=w5869:errorcluster[])
                    n2755 = call "configuration.vi"("command"="get") -> ("config out"=w5852:T13)  [unwired: 2 in, 1 out]
                    n2756 = call "tempconfigAI.vi"("command"="get") -> ("Temp Config out"=w5858:T28)  [unwired: 1 in]
                    n2757 = Unbundle By Name(w5852) -> ("Device 1 sampleclock out"=w5849:tag, "Device 1 Starttrigger out"=w5848:tag)
                    n2758 = Unbundle By Name(w5858) -> ("AI"=w5859:refnum<k21>, "E_AI"=w5860:errorcluster)
                    n2759 = for {
                      tunnel: w5870 -> [w5875] mode=indexing
                      tunnel: w5869 -> [w5874] mode=indexing
                      tunnel: [w5873] -> w5865 mode=indexing
                      n2760 = call <vilib>:"DAQmx Stop Task.vi"("task/channels in"=w5875, "error in"=w5874) -> ("task out"=w5876:refnum<k21>, "error out"=w5877:errorcluster)  [unwired: 12 in]
                      n2761 = call <vilib>:"DAQmx Clear Task.vi"("task in"=w5876, "error in"=w5877) -> ("error out"=w5873:errorcluster)  [unwired: 13 in]
                    }
                    n2762 = call <vilib>:"DAQmx Stop Task.vi"("task/channels in"=w5859, "error in"=w5860) -> ("task out"=w5856:refnum<k21>, "error out"=w5855:errorcluster)  [unwired: 12 in]
                    n2763 = call <vilib>:"DAQmx Disconnect Terminals.vi"("source terminal"=tag "/Dev1/ai/SampleClock", "destination terminal"=w5849) -> ("error out"=w5846:errorcluster)  [unwired: 13 in]
                    n2764 = call <vilib>:"DAQmx Clear Task.vi"("task in"=w5856, "error in"=w5855) -> ("error out"=w5854:errorcluster)  [unwired: 13 in]
                    n2765 = call "tempconfigAO.vi"("command"="get") -> ("Temp Config out"=w5866:T27)  [unwired: 1 in]
                    n2766 = Bundle By Name(cluster=w5866, "E_AO"=w5865) -> (w5864:T27)
                    n2767 = call "tempconfigAI.vi"("command"="get") -> ("Temp Config out"=w5862:T28)  [unwired: 1 in]
                    n2768 = Bundle By Name(cluster=w5862, "E_AI"=w5854) -> (w5853:T28)
                    n2769 = call "tempconfigAO.vi"("Temp Config in"=w5864, "command"="set") -> ()  [unwired: 1 out]
                    n2770 = call <vilib>:"DAQmx Disconnect Terminals.vi"("source terminal"=tag "/Dev1/ai/StartTrigger", "destination terminal"=w5848, "error in"=w5846) -> ()  [unwired: 12 in, 1 out]
                    n2771 = call "tempconfigAI.vi"("Temp Config in"=w5853, "command"="set") -> ()  [unwired: 1 out]
                  }
                  frame #5 {
                    w5880 = T23 4 items=["no dialog", "OK message", "continue or stop message", "OK message + warnings", "continue/stop + warnings"] ("type of dialog (OK msg:1)")
                    n2772 = call "displayerrors.vi"() -> ("error IO"=w5879:errorcluster)
                    n2773 = call "zeropatch.vi"() -> ()  [unwired: 12 in]
                    n2774 = call <vilib>:"Simple Error Handler.vi"("type of dialog (OK msg:1)"=w5880, "error in (no error)"=w5879) -> ("error out"=w5878:errorcluster)  [unwired: 3 in, 4 out]
                    n2775 = call <vilib>:"Clear Errors.vi"("error in (no error)"=w5878) -> ()  [unwired: 5 in, 2 out]
                  }
                }
              }
            }
          }
          event "readpatch": Value Change {
            n2776 = event-data() -> ()  [unwired: 1 in, 6 out]
            n2777 = case shown="True" "sealtest 2" {
              frame False {
              }
              frame True {
                n2778 = stacked-sequence {
                  seq-local: [w5882 _ _ _ _ _] -> [_ w5915 _ w5967 _ _]
                  frame #0 {
                    n2779 = stacked-sequence {
                      tunnel: [_ w5894 _] -> w5882
                      frame #0 {
                        n2780 = call "2pparameters.vi"("command"="get") -> ("params out"=w5887:T12)  [unwired: 1 in]
                        n2781 = Unbundle By Name(w5887) -> ("autoshutter"=w5888:bool)
                        n2782 = local read "OCchecked?"() -> (w5885:bool)
                        n2783 = call "sealtestwfparams.vi"("command"="set") -> ()  [unwired: 6 in, 1 out]
                        n2784 = case shown="False" w5885 {
                          frame False {
                            n2785 = One Button Dialog(message="Is the OC gain correct?", button name ("OK")="ok") -> (true=w5889:bool)
                            n2786 = local write "OCchecked?"(w5889) -> ()
                          }
                          frame True {
                          }
                        }
                        n2787 = case shown="True" w5888 {
                          frame False {
                          }
                          frame True {
                            n2788 = call "shuttercontrol.vi"("command"="close") -> ()  [unwired: 1 in, 1 out]
                          }
                        }
                        n2789 = call "allAI-temp.vi"("command"=enum16{"get", "set", "clear", "append"}."clear") -> ()  [unwired: 3 in, 2 out]
                      }
                      frame #1 {
                        n2790 = call "sealtestwfparams.vi"("command"="get") -> ("Params out"=w5900:T25)  [unwired: 6 in]
                        n2791 = Unbundle By Name(w5900) -> ("AO parameters"=w5898:T1)
                        "AO parameters 3" <- w5898
                        n2792 = Index Array(array=w5898, index=0) -> (element=w5897:T26)
                        n2793 = call "generateRampedSquareWave_fromAOparameters.vi"("AO params"=w5897) -> ("Waveform"=w5893:waveform(dbl), "wflength"=w5894:i32)
                        "Waveform Graph 2" <- w5893
                        "wflength 2" <- w5894
                        n2794 = Build Array(w5893) -> (w5896:waveform(dbl)[])
                        n2795 = call "waveformssealtestbuffer.vi"("AO wf in"=w5896, "command"="set") -> ()  [unwired: 1 out]
                      }
                      frame #2 {
                        n2796 = local read "Vholding (mV)"() -> (w5903:sgl)
                        n2797 = local read "Current Clamp"() -> (w5909:bool)
                        n2798 = local read "Voltage Clamp"() -> (w5908:bool)
                        n2799 = local read "OCgain"() -> (w5904:sgl)
                        n2800 = local read "CC_ICgain"() -> (w5907:dbl)
                        n2801 = local read "holdon"() -> (w5902:bool)
                        n2802 = call "patchparameters.vi"("command"="get") -> ("Params out"=w5911:T15)  [unwired: 1 in]
                        n2803 = Bundle By Name(cluster=w5911, "VC"=w5908, "CC"=w5909, "CC_icg (pA/mv)"=w5907, "VC_icg (mV/mV)"=10.0, "OCG (mV/pA)"=w5904, "OVG (mV/mV)"=0.1, "Vhold (mV)"=w5903, "holdon"=w5902) -> (w5910:T15)
                        n2804 = call "patchparameters.vi"("Params in"=w5910, "command"="set") -> ()  [unwired: 1 out]
                      }
                    }
                  }
                  frame #1 {
                    w5914 = 2
                    n2805 = call "patchparameters.vi"("command"="get") -> ("Params out"=w5922:T15)  [unwired: 1 in]
                    n2806 = Unbundle By Name(w5922) -> ("holdon"=w5921:bool, "Vhold (mV)"=w5920:sgl, "CC_icg (pA/mv)"=w5928:sgl, "CC"=w5926:bool, "VC_icg (mV/mV)"=w5927:sgl)
                    n2807 = Select(t=w5928, s=w5926, f=w5927) -> (s? t:f=w5929:sgl)
                    n2808 = To Single Precision Float(number=0.001 ("y")) -> (single precision float=w5930:sgl)
                    n2809 = Compound Arithmetic op=MULTIPLY(w5920, w5929, w5930) -> (w5924:sgl)
                    n2810 = case shown="False" w5921 {
                      tunnel: w5924 -> [_ w5942]
                      tunnel: [0.0 w5942] -> w5917
                      frame False {
                      }
                      frame True {
                      }
                    }
                    n2811 = Greater Than 0?(x=w5914) -> (x > 0?=w5916:bool)
                    n2812 = case shown="True" w5916 {
                      tunnel: w5915 -> [_ w5931]
                      tunnel: w5914 -> [_ w5934]
                      frame False {
                      }
                      frame True {
                        n2813 = Initialize Array(sgl 0.0 ("element"), w5934, w5931) -> (w5932:sgl[][])
                        n2814 = call "allAI-temp.vi"("array in"=w5932, "command"=enum16{"get", "set", "clear", "append"}."set") -> ()  [unwired: 2 in, 2 out]
                      }
                    }
                    n2815 = flat-sequence {
                      tunnel: w5915 -> [w5938]
                      tunnel: w5915 -> [w5937]
                      tunnel: [w5937] -> w5919
                      tunnel: [w5936] -> w5918
                      tunnel: w5917 -> [w5936]
                      tunnel: w5919 -> [w5940]
                      tunnel: w5918 -> [w5939]
                      frame #0 {
                        n2816 = call "prepAI_sealtest.vi"("samples per channel"=w5938) -> ()  [unwired: 2 in]
                      }
                      frame #1 {
                        n2817 = call "prepAO_sealtest.vi"("Vhold"=w5939, "samples per channel"=w5940) -> ()  [unwired: 1 in]
                      }
                    }
                  }
                  frame #2 {
                    n2818 = stacked-sequence {
                      frame #0 {
                        n2819 = call "tempconfigAO.vi"("command"="get") -> ("Temp Config out"=w5946:T27)  [unwired: 1 in]
                        n2820 = Unbundle By Name(w5946) -> ("AO"=w5947:refnum<k21>[], "E_AO"=w5948:errorcluster[])
                        n2821 = for {
                          tunnel: w5947 -> [w5956] mode=indexing
                          tunnel: w5948 -> [w5955] mode=indexing
                          tunnel: [w5954] -> w5950 mode=indexing
                          tunnel: [w5953] -> w5951 mode=indexing
                          n2822 = call <vilib>:"DAQmx Start Task.vi"("task/channels in"=w5956, "error in"=w5955) -> ("task out"=w5954:refnum<k21>, "error out"=w5953:errorcluster)  [unwired: 12 in]
                        }
                        n2823 = call "tempconfigAO.vi"("command"="get") -> ("Temp Config out"=w5949:T27)  [unwired: 1 in]
                        n2824 = Bundle By Name(cluster=w5949, "AO"=w5950, "E_AO"=w5951) -> (w5952:T27)
                        n2825 = call "tempconfigAO.vi"("Temp Config in"=w5952, "command"="set") -> ()  [unwired: 1 out]
                      }
                      frame #1 {
                        n2826 = call "tempconfigAI.vi"("command"="get") -> ("Temp Config out"=w5958:T28)  [unwired: 1 in]
                        n2827 = Unbundle By Name(w5958) -> ("AI"=w5963:refnum<k21>, "E_AI"=w5964:errorcluster)
                        n2828 = call <vilib>:"DAQmx Start Task.vi"("task/channels in"=w5963, "error in"=w5964) -> ("task out"=w5965:refnum<k21>, "error out"=w5966:errorcluster)  [unwired: 12 in]
                        n2829 = call "tempconfigAI.vi"("command"="get") -> ("Temp Config out"=w5960:T28)  [unwired: 1 in]
                        n2830 = Bundle By Name(cluster=w5960, "AI"=w5965, "E_AI"=w5966) -> (w5962:T28)
                        n2831 = call "tempconfigAI.vi"("Temp Config in"=w5962, "command"="set") -> ()  [unwired: 1 out]
                      }
                    }
                  }
                  frame #3 {
                    n2832 = while {
                      tunnel: w5967 -> [w5968]
                      stop <- w5969 stop-if-true
                      n2833 = local read "sealtest 2"() -> (w5972:bool)
                      n2834 = Not(x=w5972) -> (.not. x?=w5971:bool)
                      n2835 = case shown="False" w5971 {
                        tunnel: w5968 -> [w5973 _]
                        frame False {
                          n2836 = stacked-sequence {
                            seq-local: [_ _ _ w6012 _ _] -> [_ _ _ _ w6068 _]
                            seq-local: [w5974 _ _ _ _ _] -> [_ w5983 _ w6005 w6057 w6088]
                            tunnel: w5973 -> [_ _ w5991 _ w6056 _]
                            frame #0 {
                              n2837 = call "patchparameters.vi"("command"="get") -> ("Params out"=w5981:T15)  [unwired: 1 in]
                              n2838 = local read "Vholding (mV)"() -> (w5978:sgl)
                              n2839 = Unbundle By Name(w5981) -> ("Vhold (mV)"=w5977:sgl, "holdon"=w5980:bool)
                              n2840 = local read "holdon"() -> (w5979:bool)
                              n2841 = Not Equal?(x=w5978, y=w5977) -> (x != y?=w5976:bool)
                              n2842 = Not Equal?(x=w5980, y=w5979) -> (x != y?=w5975:bool)
                              n2843 = Or(x=w5976, y=w5975) -> (x .or. y?=w5974:bool)
                            }
                            frame #1 {
                              n2844 = case shown="True" w5983 {
                                frame False {
                                }
                                frame True {
                                n2845 = local read "Vholding (mV)"() -> (w5986:sgl)
                                n2846 = local read "holdon"() -> (w5984:bool)
                                n2847 = call "patchparameters.vi"("command"="get") -> ("Params out"=w5987:T15)  [unwired: 1 in]
                                n2848 = Bundle By Name(cluster=w5987, "Vhold (mV)"=w5986, "holdon"=w5984) -> (w5985:T15)
                                n2849 = call "patchparameters.vi"("Params in"=w5985, "command"="set") -> ()  [unwired: 1 out]
                                }
                              }
                            }
                            frame #2 {
                              n2850 = call "tempconfigAI.vi"("command"="get") -> ("Temp Config out"=w6001:T28)  [unwired: 1 in]
                              n2851 = Unbundle By Name(w6001) -> ("AI"=w6000:refnum<k21>, "E_AI"=w5999:errorcluster)
                              n2852 = call-poly <vilib>:"DAQmx Read.vi"("task/channels in"=w6000, "number of samples per channel"=w5991, "timeout"=10.0, "error in"=w5999) -> ("task out"=w5995:refnum<k21>, "data"=w5992:i16[][], "error out"=w6004:errorcluster)  [unwired: 9 in]
                              n2853 = call "tempconfigAI.vi"("command"="get") -> ("Temp Config out"=w5996:T28)  [unwired: 1 in]
                              n2854 = Bundle By Name(cluster=w5996, "AI"=w5995, "E_AI"=w6004) -> (w6003:T28)
                              n2855 = To Single Precision Float(number=w5992) -> (single precision float=w5994:sgl[][])
                              n2856 = call "tempconfigAI.vi"("Temp Config in"=w6003, "command"="set") -> ()  [unwired: 1 out]
                              n2857 = call "allAI-temp.vi"("array in"=w5994, "command"=enum16{"get", "set", "clear", "append"}."set") -> ()  [unwired: 2 in, 2 out]
                            }
                            frame #3 {
                              n2858 = case shown="True" w6005 {
                                frame False {
                                }
                                frame True {
                                n2859 = call "tempconfigAO.vi"("command"="get") -> ("Temp Config out"=w6045:T27)  [unwired: 1 in]
                                n2860 = Unbundle By Name(w6045) -> ("AO"=w6044:refnum<k21>[], "E_AO"=w6043:errorcluster[])
                                n2861 = call "tempconfigAI.vi"("command"="get") -> ("Temp Config out"=w6032:T28)  [unwired: 1 in]
                                n2862 = Unbundle By Name(w6032) -> ("AI"=w6033:refnum<k21>, "E_AI"=w6034:errorcluster)
                                n2863 = for {
                                tunnel: w6044 -> [w6049] mode=indexing
                                tunnel: w6043 -> [w6048] mode=indexing
                                tunnel: [w6047] -> w6039 mode=indexing
                                n2864 = call <vilib>:"DAQmx Stop Task.vi"("task/channels in"=w6049, "error in"=w6048) -> ("task out"=w6050:refnum<k21>, "error out"=w6051:errorcluster)  [unwired: 12 in]
                                n2865 = call <vilib>:"DAQmx Clear Task.vi"("task in"=w6050, "error in"=w6051) -> ("error out"=w6047:errorcluster)  [unwired: 13 in]
                                }
                                n2866 = call <vilib>:"DAQmx Stop Task.vi"("task/channels in"=w6033, "error in"=w6034) -> ("task out"=w6030:refnum<k21>, "error out"=w6029:errorcluster)  [unwired: 12 in]
                                n2867 = call <vilib>:"DAQmx Clear Task.vi"("task in"=w6030, "error in"=w6029) -> ("error out"=w6028:errorcluster)  [unwired: 13 in]
                                n2868 = call "tempconfigAO.vi"("command"="get") -> ("Temp Config out"=w6040:T27)  [unwired: 1 in]
                                n2869 = Bundle By Name(cluster=w6040, "E_AO"=w6039) -> (w6038:T27)
                                n2870 = call "tempconfigAI.vi"("command"="get") -> ("Temp Config out"=w6036:T28)  [unwired: 1 in]
                                n2871 = Bundle By Name(cluster=w6036, "E_AI"=w6028) -> (w6027:T28)
                                n2872 = call "tempconfigAO.vi"("Temp Config in"=w6038, "command"="set") -> ()  [unwired: 1 out]
                                n2873 = call "tempconfigAI.vi"("Temp Config in"=w6027, "command"="set") -> ()  [unwired: 1 out]
                                }
                              }
                              n2874 = call "allAI-temp.vi"("command"=enum16{"get", "set", "clear", "append"}."get") -> ("array out"=w6009:sgl[][])  [unwired: 3 in, 1 out]
                              n2875 = call "tempconfigAI.vi"("command"="get") -> ("Temp Config out"=w6022:T28)  [unwired: 1 in]
                              n2876 = call "tempconfigAI.vi"("command"="get") -> ("Temp Config out"=w6024:T28)  [unwired: 1 in]
                              n2877 = Unbundle By Name(w6022) -> ("header"=w6020:dbl[])
                              n2878 = Unbundle By Name(w6024) -> ("header"=w6026:dbl[])
                              n2879 = Index Array(array=w6009, index (row) #1=1 ("index (row)"), index (row) #2=0 ("index (row)")) -> (element #1=w6007:sgl[], element #2=w6006:sgl[])  [unwired: 2 in]
                              n2880 = local read "OCgain"() -> (w6014:sgl)
                              n2881 = call "Unscaledtoscaled.vi"("Unscaled Data"=w6007, "Header Information"=w6020) -> ("Array"=w6019:sgl[])  [unwired: 1 in]
                              n2882 = call "Unscaledtoscaled.vi"("Unscaled Data"=w6006, "Header Information"=w6026) -> ("Array"=w6023:sgl[])  [unwired: 1 in]
                              n2883 = Multiply(x=w6019, y=0.1) -> (x*y=w6016:dbl[])
                              n2884 = Divide(x=w6023, y=w6014) -> (x/y=w6015:sgl[])
                              n2885 = Build Array(w6016, w6015) -> (w6018:dbl[][])
                              n2886 = Multiply(x=w6018, y=1000.0) -> (x*y=w6012:dbl[][])
                              "Patch readout 2" <- w6012
                            }
                            frame #4 {
                              n2887 = case shown="True" w6057 {
                                tunnel: w6056 -> [_ w6069]
                                frame False {
                                }
                                frame True {
                                n2888 = call "patchparameters.vi"("command"="get") -> ("Params out"=w6073:T15)  [unwired: 1 in]
                                n2889 = Unbundle By Name(w6073) -> ("holdon"=w6072:bool, "Vhold (mV)"=w6071:sgl, "CC_icg (pA/mv)"=w6079:sgl, "CC"=w6077:bool, "VC_icg (mV/mV)"=w6078:sgl)
                                n2890 = Select(t=w6079, s=w6077, f=w6078) -> (s? t:f=w6080:sgl)
                                n2891 = To Single Precision Float(number=0.001 ("y")) -> (single precision float=w6081:sgl)
                                n2892 = Compound Arithmetic op=MULTIPLY(w6071, w6080, w6081) -> (w6075:sgl)
                                n2893 = case shown="True" w6072 {
                                tunnel: w6075 -> [_ w6086]
                                tunnel: [0.0 w6086] -> w6070
                                frame False {
                                }
                                frame True {
                                }
                                }
                                n2894 = flat-sequence {
                                tunnel: w6069 -> [w6082]
                                tunnel: w6070 -> [w6084]
                                tunnel: w6069 -> [w6083]
                                frame #0 {
                                n2895 = call "prepAI_sealtest.vi"("samples per channel"=w6082) -> ()  [unwired: 2 in]
                                }
                                frame #1 {
                                n2896 = call "prepAO_sealtest.vi"("Vhold"=w6084, "samples per channel"=w6083) -> ()  [unwired: 1 in]
                                }
                                }
                                }
                              }
                              n2897 = call "sealtestwfparams.vi"("command"="get") -> ("Params out"=w6062:T25)  [unwired: 6 in]
                              n2898 = Unbundle By Name(w6062) -> ("AO parameters"=w6063:T1)
                              n2899 = Index Array(array=w6063, index=0) -> (element=w6065:T26)
                              n2900 = Unbundle By Name(w6065) -> ("Cycles"=w6060:dbl, "Start amplitude (V)"=w6059:dbl, "Sampling frequency (Hz)"=w6058:dbl)
                              n2901 = local read "fitpoints"() -> (w6066:dbl)
                              n2902 = script code="V=data(1,:);\nI=data(2,:);\ntres=mean(V);\nspc=(nsamp./ncyc);\nV=V(spc+1:end-spc);\nI=I(spc+1:end-spc);\ndV=mean(V(V>tres))-mean(V(V<tres))\nIcyc=reshape(I,[spc ncyc-2]);\nIcyc=Icyc';\nIcyc=mean(Icyc,1);\ndIss=mean(Icyc(floor(spc*0.15):floor(spc/2)-2))-mean(Icyc(spc*0.65:spc-2))\nRm=dV*1e3/dIss;\n[maxi,ind]=max(Icyc);\nIfit=Icyc(ind+1:ind+1+points-1)-0.5*(mean(Icyc(floor(spc*0.15):floor(spc/2)-2))+mean(Icyc(spc*0.65:spc-2)))\nt=(3:points-1+3)./srate*1000;\nt=t';\nIfit=Ifit';\nc=fit(t,Ifit, 'exp1');\ncoeffs=coeffvalues(c);\nIa=coeffs(1);\nRa=dV*1e3./Ia/2;\ntau=-1./coeffs(2);\ncap=tau/Ra*1000;"("data"=w6068, "nsamp"=w6056, "ncyc"=w6060, "maxV"=w6059, "points"=w6066, "srate"=w6058) -> ("cap"=w6055:dbl, "Ra"=w6054:dbl, "Icyc"=w6053:dbl[], "Rm"=w6052:dbl)  [unwired: 1 in, 1 out]
                              n2903 = local read "set as Rp?"() -> (w6067:bool)
                              n2904 = local write "Cmembrane"(w6055) -> ()
                              n2905 = local write "Rmembrane (MOhm)"(w6052) -> ()
                              n2906 = local write "Racces (MOhm)"(w6054) -> ()
                              n2907 = case shown="True" w6067 {
                                tunnel: w6052 -> [_ w6087]
                                frame False {
                                }
                                frame True {
                                n2908 = local write "Rpipette (MOhm)"(w6087) -> ()
                                }
                              }
                              n2909 = local write "Ifit"(w6053) -> ()
                            }
                            frame #5 {
                              n2910 = local read "set as Rp?"() -> (w6089:bool)
                              n2911 = case shown="True" w6088 {
                                frame False {
                                }
                                frame True {
                                n2912 = stacked-sequence {
                                frame #0 {
                                n2913 = call "tempconfigAO.vi"("command"="get") -> ("Temp Config out"=w6096:T27)  [unwired: 1 in]
                                n2914 = Unbundle By Name(w6096) -> ("AO"=w6095:refnum<k21>[], "E_AO"=w6094:errorcluster[])
                                n2915 = for {
                                tunnel: w6095 -> [w6103] mode=indexing
                                tunnel: w6094 -> [w6102] mode=indexing
                                tunnel: [w6101] -> w6092 mode=indexing
                                tunnel: [w6100] -> w6091 mode=indexing
                                n2916 = call <vilib>:"DAQmx Start Task.vi"("task/channels in"=w6103, "error in"=w6102) -> ("task out"=w6101:refnum<k21>, "error out"=w6100:errorcluster)  [unwired: 12 in]
                                }
                                n2917 = call "tempconfigAO.vi"("command"="get") -> ("Temp Config out"=w6093:T27)  [unwired: 1 in]
                                n2918 = Bundle By Name(cluster=w6093, "AO"=w6092, "E_AO"=w6091) -> (w6090:T27)
                                n2919 = call "tempconfigAO.vi"("Temp Config in"=w6090, "command"="set") -> ()  [unwired: 1 out]
                                }
                                frame #1 {
                                n2920 = call "tempconfigAI.vi"("command"="get") -> ("Temp Config out"=w6105:T28)  [unwired: 1 in]
                                n2921 = Unbundle By Name(w6105) -> ("AI"=w6110:refnum<k21>, "E_AI"=w6111:errorcluster)
                                n2922 = call <vilib>:"DAQmx Start Task.vi"("task/channels in"=w6110, "error in"=w6111) -> ("task out"=w6112:refnum<k21>, "error out"=w6113:errorcluster)  [unwired: 12 in]
                                n2923 = call "tempconfigAI.vi"("command"="get") -> ("Temp Config out"=w6107:T28)  [unwired: 1 in]
                                n2924 = Bundle By Name(cluster=w6107, "AI"=w6112, "E_AI"=w6113) -> (w6109:T28)
                                n2925 = call "tempconfigAI.vi"("Temp Config in"=w6109, "command"="set") -> ()  [unwired: 1 out]
                                }
                                }
                                }
                              }
                              n2926 = case shown="True" w6089 {
                                frame False {
                                }
                                frame True {
                                n2927 = local write "set as Rp?"(FALSE ("set as Rp?")) -> ()
                                }
